vi "Test Process In Process Loop True when Uninitialized.vi"(8 "error in (no error)":errorcluster, 11 "Process Test In":refnum<class "Process Dev Test.lvclass">) -> (0 "error out":errorcluster, 3 "Process Test Out":refnum<class "Process Dev Test.lvclass">)   [LabVIEW 2020, in "Process Dev Test.lvclass"]
uses:
  Process Dev Test.lvclass
  Process Dev Test.lvclass/Process Dev Test.ctl
  source/Framework/Process/Process.lvclass
  7f55a702-0c1c-4b33-b254-360e9ddefc0b.vi
  source/Framework/Process/Public/Lifecycle/API Mode.ctl
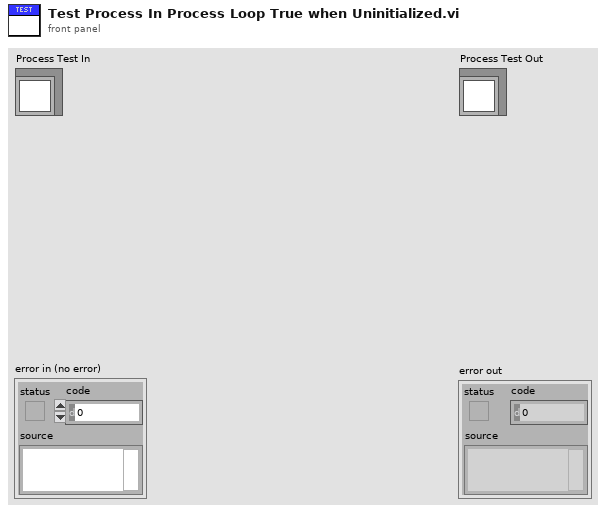
[diagram p1: front panel]
types:
  T1 = typedef "Process.lvclass/API Mode.ctl" = enum16{"Send Message", "Handle Message"}
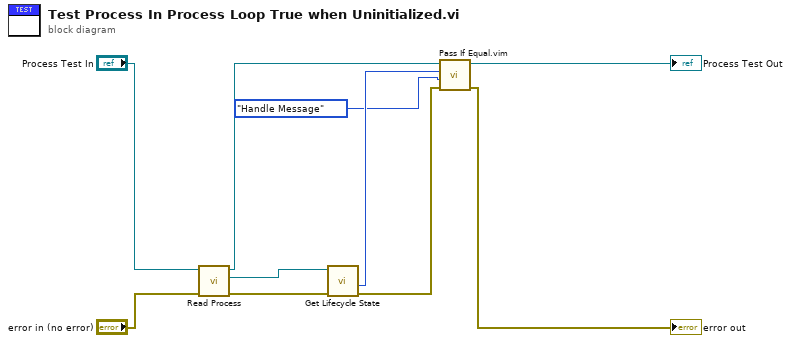
[diagram p0: block diagram]
diagram:
  n1 = call "Read Process.vi"("error in (no error)"="error in (no error)", "Process Test in"="Process Test In") -> ("error out"=w5:errorcluster, "Process.lvclass"=w6:refnum<class "Process.lvclass">, "Process Test out"=w3:refnum<class "Process Dev Test.lvclass">)  [unwired: 7 in]
  n2 = call "Get Lifecycle State.vi"("error in (no error)"=w5, "Process In"=w6) -> ("error out"=w9:errorcluster, "API Mode"=w2:T1)  [unwired: 6 in, 2 out]
  n3 = call "Pass If Equal.vim"("error in (no error)"=w9, "Actual"=API_Mode."Handle Message" ("API Mode"), "Expected"=w2, "LUnit Test Case In"=w3) -> ("error out"=→"error out":errorcluster, "LUnit Test Case Out"=→"Process Test Out":refnum<class "Process Dev Test.lvclass">)  [unwired: 6 in]
